vi "FindNextTarget.vi"(8 "error in (no error)":errorcluster, 9 "CurPos":i32, 10 "Runlist":i32[][](array[numeric]), 11 "RunsDone":i32[][](array[numeric])) -> (0 "error out":errorcluster, 1 "NextPos":i32)   [LabVIEW 2013]
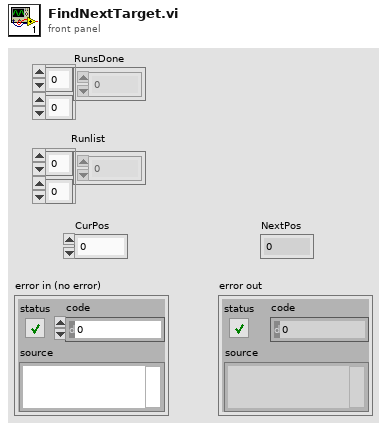
[diagram p1: front panel]
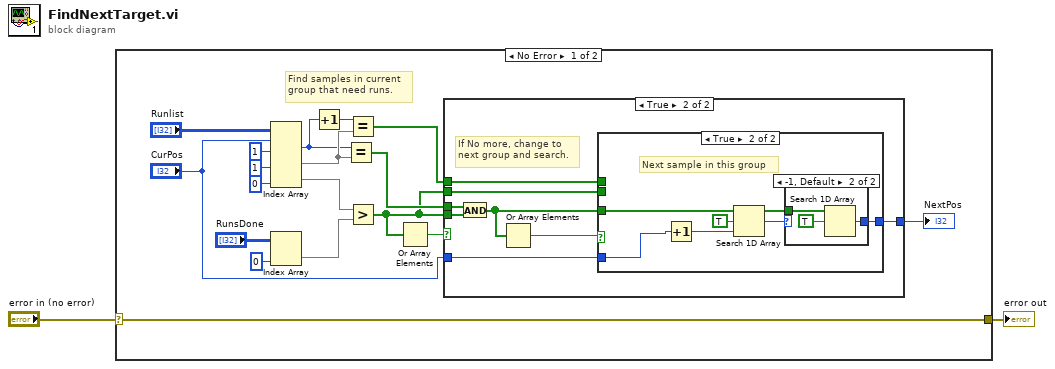
[diagram p0: block diagram]
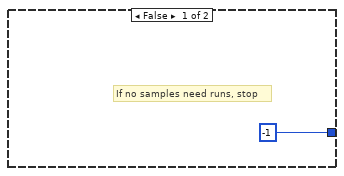
[diagram p2: hidden frame]
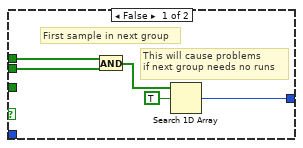
[diagram p3: hidden frame]
diagram:
  n1 = case shown="No Error" "error in (no error)" {
    selector: "error in (no error)" -> [w12 w45]
    tunnel: [w12 w45] -> w1
    frame No Error {
      # "Find samples in current\ngroup that need runs."
      n2 = Index Array(array="Runlist", index (row) #1="CurPos", index (col) #1=1 ("disabled index (col)"), index (col) #2=1 ("index (col)"), index (col) #3=0 ("disabled index (col)")) -> (element #1=w5:i32, element #2=w7:i32[], element #3=w9:i32[])  [unwired: 2 in]
      n3 = Index Array(array="RunsDone", index (col)=0 ("disabled index (col)")) -> (element=w16:i32[])  [unwired: 1 in]
      n4 = Increment(x=w5) -> (x+1=w6:i32)
      n5 = Equal?(x=w5, y=w7) -> (x = y?=w14:bool[])
      n6 = Equal?(x=w6, y=w7) -> (x = y?=w4:bool[])
      n7 = Greater?(x=w9, y=w16) -> (0:w3:bool[])
      n8 = Or Array Elements(Boolean array=w3) -> (logical OR=w11:bool)
      n9 = case shown="True" w11 {
        tunnel: [-1 ("index of element") w29] -> w20
        tunnel: w3 -> [_ w28]
        tunnel: w14 -> [_ w27]
        tunnel: "CurPos" -> [_ w24]
        tunnel: w4 -> [_ w23]
        tunnel: w3 -> [_ w22]
        frame False {
          # "If no samples need runs, stop"
        }
        frame True {
          # "If No more, change to\nnext group and search."
          n10 = And(x=w27, y=w28) -> (x .and. y?=w26:bool[])
          n11 = Or Array Elements(Boolean array=w26) -> (logical OR=w25:bool)
          n12 = case shown="True" w25 {
            tunnel: [w30 w40] -> w29
            tunnel: w26 -> [_ w37]
            tunnel: w24 -> [_ w36]
            tunnel: w23 -> [w34 _]
            tunnel: w22 -> [w33 _]
            frame False {
              # "This will cause problems \nif next group needs no runs"
              # "First sample in next group"
              n13 = And(x=w34, y=w33) -> (x .and. y?=w31:bool[])
              n14 = Search 1D Array(1D array=w31, element=TRUE) -> (index of element=w30:i32)  [unwired: 1 in]
            }
            frame True {
              # "Next sample in this group"
              n15 = Increment(x=w36) -> (x+1=w35:i32)
              n16 = Search 1D Array(1D array=w37, element=TRUE, start index (0)=w35) -> (index of element=w39:i32)
              n17 = case shown="-1, Default" w39 {
                selector: w39 -> [w41 _]
                tunnel: [w41 w43] -> w40
                tunnel: w37 -> [_ w42]
                frame 0..133 {
                }
                frame -1, Default {
                  n18 = Search 1D Array(1D array=w42, element=TRUE) -> (index of element=w43:i32)  [unwired: 1 in]
                }
              }
            }
          }
        }
      }
      "NextPos" <- w20
    }
    frame Error {
    }
  }
  "error out" <- w1
